vi "Write JSON reader.vi"(8 "error in (no error)":errorcluster, 10 "JSON reader.lvclass":refnum<class "JSON reader.lvclass">, 11 "Interface in":refnum<class "Interface.lvclass">) -> (0 "error out":errorcluster, 3 "Interface out":refnum<class "Interface.lvclass">)   [LabVIEW 2018, in "Interface.lvclass"]
uses:
  Interface.lvclass
  JSON reader/JSON reader.lvclass
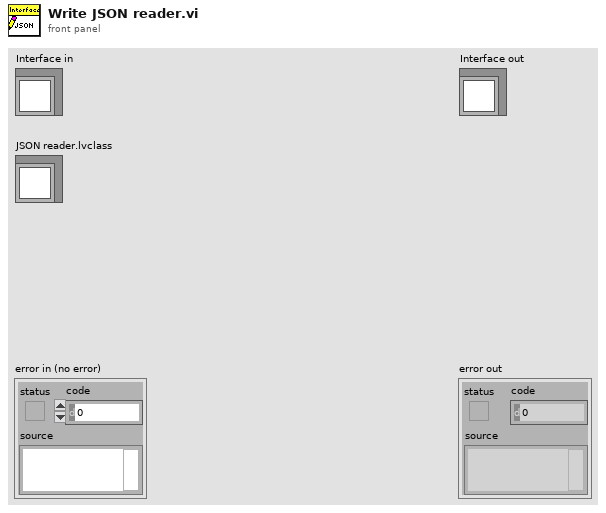
[diagram p1: front panel]
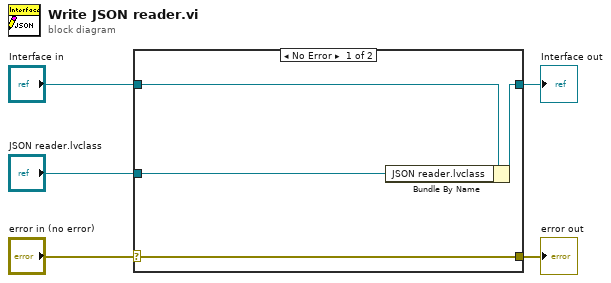
[diagram p0: block diagram]
diagram:
  n1 = case shown="No Error" "error in (no error)" {
    selector: "error in (no error)" -> [w9 w10]
    tunnel: [w9 w10] -> w4
    tunnel: [w7 w11] -> w2
    tunnel: "Interface in" -> [w8 w11]
    tunnel: "JSON reader.lvclass" -> [w6 _]
    frame No Error {
      n2 = Bundle By Name(cluster=w8, "JSON reader.lvclass"=w6) -> (w7:refnum<class "Interface.lvclass">)
    }
    frame Error {
    }
  }
  "error out" <- w4
  "Interface out" <- w2
